vi "close connection.vi"(8 "error in (no error)":errorcluster, 11 "Tektronix RSA5106A in":refnum<class "Tektronix RSA5106A.lvclass">) -> (0 "error out":errorcluster, 3 "Tektronix RSA5106A out":refnum<class "Tektronix RSA5106A.lvclass">)   [LabVIEW 2013, in "Tektronix RSA5106A.lvclass"]
uses:
  Tektronix RSA5106A.lvclass
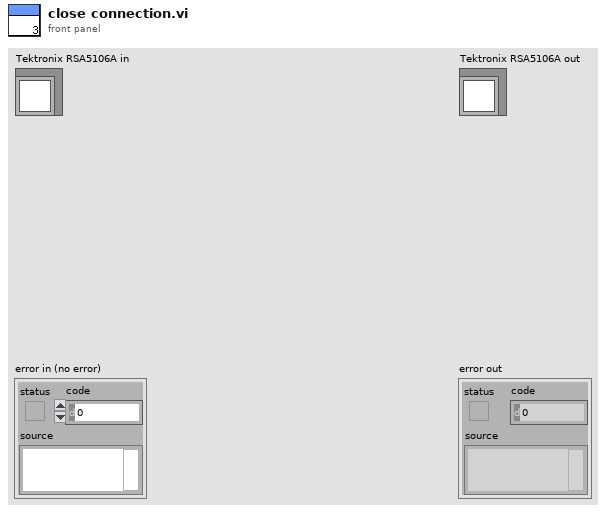
[diagram p1: front panel]
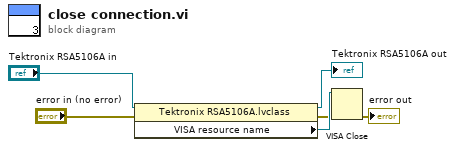
[diagram p0: block diagram]
diagram:
  n1 = property class="Tektronix RSA5106A.lvclass"(reference="Tektronix RSA5106A in", error in="error in (no error)") -> (reference out=→"Tektronix RSA5106A out":refnum<class "Tektronix RSA5106A.lvclass">, error out=w1:errorcluster, "VISA resource name"=w5:refnum<visa-resource-name>)
  n2 = VISA Close(VISA resource name=w5, error in (no error)=w1) -> (error out=→"error out":errorcluster)
